vi "ComicCleaner.vi"() -> ()   [LabVIEW 2022 SP3]
uses:
  TypeDefs/Main States.ctl
  TypeDefs/Tag Cmd.ctl
panel:
  in  "Clean Filename?":bool=TRUE
  out "Total":i32
  out "Progress":i32(slide) max=10 scale=0.0..4.0
  out "Current File":string
  in  "Directory":path
  out "Status":string
  out "Crufted Files":string[](array[string])
  in  "Single File":path
  out "Working Folder":path=path "C:/Users/Mark/Documents/Temp"
  in  "Exit":bool
  # "of"
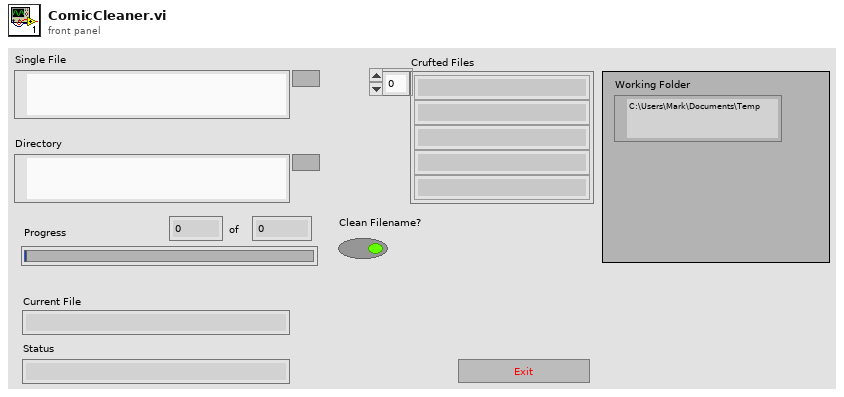
[diagram p1: front panel]
types:
  T1 = typedef "Main States.ctl" = enum16{"Init", "Clean Single", "Clean Dir", "Wait For Input", "Exit"}
  T2 = typedef "Tag Cmd.ctl" = enum16{"Init", "Get Known", "Set Known"}
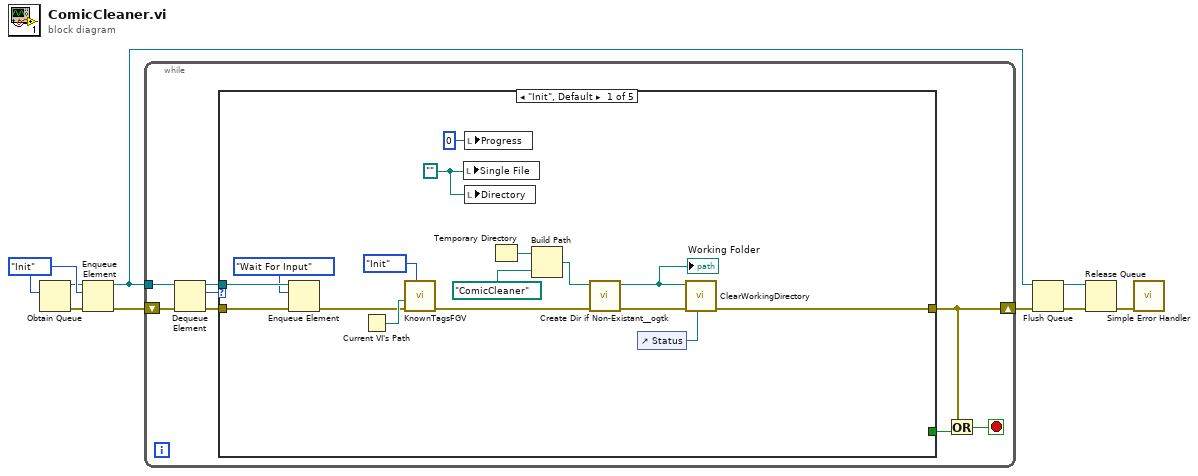
[diagram p0: block diagram]
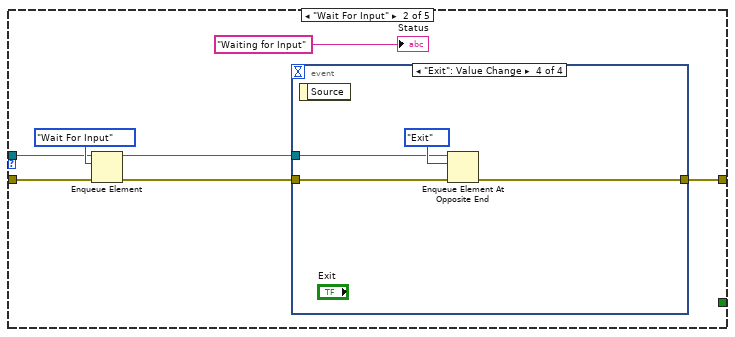
[diagram p2: hidden frame]
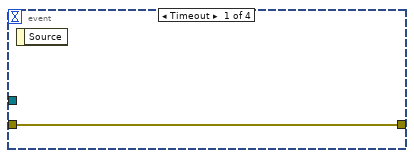
[diagram p3: hidden frame]
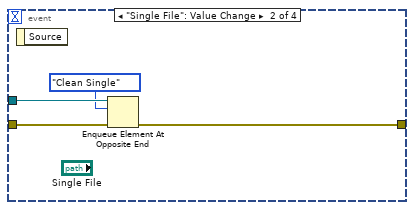
[diagram p4: hidden frame]
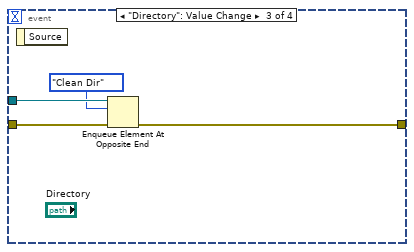
[diagram p5: hidden frame]
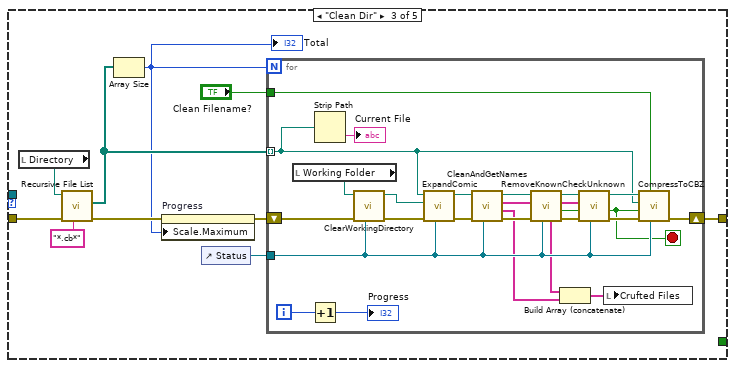
[diagram p6: hidden frame]
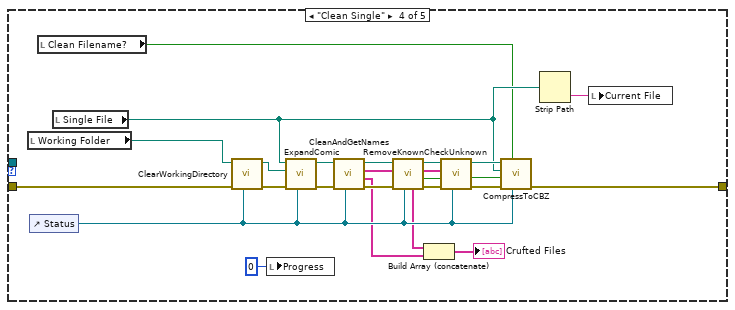
[diagram p7: hidden frame]
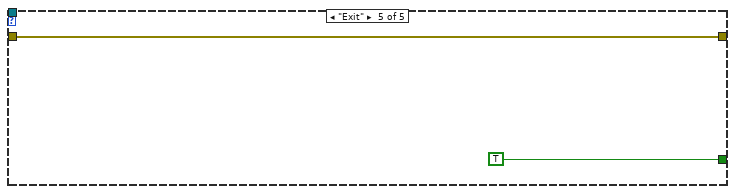
[diagram p8: hidden frame]
diagram:
  w9 = Main_States."Init" ("State")
  n1 = Obtain Queue(element data type=w9) -> (queue out=w8:refnum<queue>, error out=w7:errorcluster)  [unwired: 4 in, 1 out]
  n2 = Enqueue Element(queue=w8, element=w9, error in (no error)=w7) -> (queue out=w1:refnum<queue>, error out=w6:errorcluster)  [unwired: 1 in, 1 out]
  n3 = while {
    shift-right: [w10] -> w3
    shift-left: w6 -> [w17]
    tunnel: w1 -> [w16]
    stop <- w12 stop-if-true
    n4 = Dequeue Element(queue=w16, error in (no error)=w17) -> (queue out=w11:refnum<queue>, element=w15:T1, error out=w14:errorcluster)  [unwired: 1 in, 1 out]
    n5 = case shown="\"Init\", Default" w15 {
      tunnel: w11 -> [w29 w37 _ _ _]
      tunnel: w14 -> [w28 w36 w63 w114 w115]
      tunnel: [_ _ _ _ TRUE] -> w13
      tunnel: [w30 w40 w60 w99 w115] -> w10
      frame "Init", Default {
        w24 = path ""
        n6 = Enqueue Element(queue=w29, element=Main_States."Wait For Input" ("State"), error in (no error)=w28) -> (error out=w27:errorcluster)  [unwired: 1 in, 2 out]
        n7 = Current VI's Path() -> (path=w32:path)
        n8 = call "KnownTagsFGV.vi"("Tag Cmd"=Tag_Cmd."Init", "error in (no error)"=w27, "ini Path"=w32) -> ("error out"=w20:errorcluster)  [unwired: 7 in, 1 out]
        n9 = local write "Single File"(w24) -> ()
        n10 = local write "Progress"(u8 0 ("Progress")) -> ()
        n11 = local write "Directory"(w24) -> ()
        n12 = Temporary Directory() -> (w23:path)
        n13 = Build Path(base path=w23, name or relative path=path "ComicCleaner") -> (appended path=w21:path)
        n14 = call <userlib>:"Create Dir if Non-Existant__ogtk.vi"("error in (no error)"=w20, "Directory Path"=w21) -> ("error out"=w19:errorcluster, "dup Directory Path"=w18:path)  [unwired: 7 in, 1 out]
        "Working Folder" <- w18
        n15 = control-ref of="Status"() -> (w31:refnum<vi>)
        n16 = call "ClearWorkingDirectory.vi"("Status"=w31, "error in"=w19, "Working Path"=w18) -> ("error out"=w30:errorcluster)  [unwired: 7 in, 1 out]
      }
      frame "Wait For Input" {
        n17 = Enqueue Element(queue=w37, element=Main_States."Wait For Input" ("State"), error in (no error)=w36) -> (queue out=w34:refnum<queue>, error out=w35:errorcluster)  [unwired: 1 in, 1 out]
        n18 = event shown="[3] \"Exit\": Value Change" {
          selector: _ -> [_ _ _ _]
          dyn-events: _ -> [_ _ _ _]
          timeout: _ -> [_ _ _ _]
          tunnel: [w41 w42 w46 w50] -> w40
          tunnel: w35 -> [w41 w45 w49 w51]
          tunnel: w34 -> [_ w44 w48 w52]
          event Timeout {
            n19 = event-data() -> ()  [unwired: 1 in, 1 out]
          }
          event "Single File": Value Change {
            n20 = event-data() -> ()  [unwired: 1 in, 1 out]
            n21 = Enqueue Element At Opposite End(queue=w44, element=Main_States."Clean Single" ("State"), error in (no error)=w45) -> (error out=w42:errorcluster)  [unwired: 1 in, 2 out]
          }
          event "Directory": Value Change {
            n22 = event-data() -> ()  [unwired: 1 in, 1 out]
            n23 = Enqueue Element At Opposite End(queue=w48, element=Main_States."Clean Dir" ("State"), error in (no error)=w49) -> (error out=w46:errorcluster)  [unwired: 1 in, 2 out]
          }
          event "Exit": Value Change {
            n24 = event-data() -> ()  [unwired: 1 in, 1 out]
            n25 = Enqueue Element At Opposite End(queue=w52, element=Main_States."Exit" ("State"), error in (no error)=w51) -> (error out=w50:errorcluster)  [unwired: 1 in, 2 out]
          }
        }
        "Status" <- "Waiting for Input" ("Status")
      }
      frame "Clean Dir" {
        n26 = local read "Directory"() -> (w62:path)
        n27 = call <vilib>:"Recursive File List.vi"("pattern"="*.cb*", "error in (no error)"=w63, "Folder Path"=w62) -> ("error out"=w57:errorcluster, "All Files in Dir"=w58:path[])  [unwired: 4 in, 3 out]
        n28 = Array Size(array=w58) -> (size(s)=w55:i32)
        "Total" <- w55
        n29 = property on="Progress" class="Slide (strict)"(error in=w57, "Scale.Maximum"=w55) -> (error out=w56:errorcluster)  [unwired: 1 in, 1 out]
        n30 = control-ref of="Status"() -> (w59:refnum<vi>)
        n31 = for {
          N: w55 -> [_]
          shift-right: [w73] -> w60
          shift-left: w56 -> [w74]
          tunnel: w58 -> [w72] mode=indexing
          tunnel: w59 -> [w75]
          tunnel: "Clean Filename?" -> [w64]
          i -> [w66]
          stop <- w70 stop-if-true
          n32 = local read "Working Folder"() -> (w89:path)
          n33 = Increment(x=w66) -> (x+1=→"Progress":i32)
          n34 = Strip Path(path=w72) -> (name=→"Current File":string)  [unwired: 1 out]
          n35 = call "ClearWorkingDirectory.vi"("Status"=w75, "error in"=w74, "Working Path"=w89) -> ("error out"=w88:errorcluster, "Working Path Out"=w87:path)  [unwired: 7 in]
          n36 = call "ExpandComic.vi"("Status"=w75, "error in (no error)"=w88, "Working Dir"=w87, "Source"=w72) -> ("error out"=w85:errorcluster, "Working Dir Out"=w86:path)  [unwired: 6 in]
          n37 = call "CleanAndGetNames.vi"("Status"=w75, "error in"=w85, "Working Dir"=w86) -> ("error out"=w84:errorcluster, "Deleted files"=w68:string[], "filenames"=w83:string[], "Working Dir Out"=w82:path)  [unwired: 5 in]
          n38 = call "RemoveKnown.vi"("Status"=w75, "error in (no error)"=w84, "filenames"=w83, "Working Dir"=w82) -> ("error out"=w80:errorcluster, "Known Found?"=w79:bool, "Filenames Out"=w78:string[], "Working Dir Out"=w81:path, "Tags Removed"=w69:string[])  [unwired: 3 in]
          n39 = Build Array (concatenate)(w69, w68) -> (w67:string[])
          n40 = call "CheckUnknown.vi"("Status"=w75, "error in (no error)"=w80, "Known Found?"=w79, "filenames"=w78, "Working Dir"=w81) -> ("error out"=w76:errorcluster, "Abort?"=w70:bool, "Working Dir Out"=w77:path)  [unwired: 4 in]
          n41 = local write "Crufted Files"(w67) -> ()
          n42 = call "CompressToCBZ.vi"("Status"=w75, "Clean Filename?"=w64, "error in"=w76, "Abort?"=w70, "FormerFilename"=w72, "Working Path"=w77) -> ("error out"=w73:errorcluster)  [unwired: 4 in, 1 out]
        }
      }
      frame "Clean Single" {
        n43 = local read "Working Folder"() -> (w113:path)
        n44 = control-ref of="Status"() -> (w98:refnum<vi>)
        n45 = local read "Clean Filename?"() -> (w90:bool)
        n46 = local read "Single File"() -> (w97:path)
        n47 = call "ClearWorkingDirectory.vi"("Status"=w98, "error in"=w114, "Working Path"=w113) -> ("error out"=w112:errorcluster, "Working Path Out"=w111:path)  [unwired: 7 in]
        n48 = local write "Progress"(u8 0 ("Progress")) -> ()
        n49 = call "ExpandComic.vi"("Status"=w98, "error in (no error)"=w112, "Working Dir"=w111, "Source"=w97) -> ("error out"=w109:errorcluster, "Working Dir Out"=w110:path)  [unwired: 6 in]
        n50 = call "CleanAndGetNames.vi"("Status"=w98, "error in"=w109, "Working Dir"=w110) -> ("error out"=w108:errorcluster, "Deleted files"=w93:string[], "filenames"=w107:string[], "Working Dir Out"=w106:path)  [unwired: 5 in]
        n51 = call "RemoveKnown.vi"("Status"=w98, "error in (no error)"=w108, "filenames"=w107, "Working Dir"=w106) -> ("error out"=w104:errorcluster, "Known Found?"=w103:bool, "Filenames Out"=w102:string[], "Working Dir Out"=w105:path, "Tags Removed"=w94:string[])  [unwired: 3 in]
        n52 = Build Array (concatenate)(w94, w93) -> (→"Crufted Files":string[])
        n53 = call "CheckUnknown.vi"("Status"=w98, "error in (no error)"=w104, "Known Found?"=w103, "filenames"=w102, "Working Dir"=w105) -> ("error out"=w100:errorcluster, "Abort?"=w95:bool, "Working Dir Out"=w101:path)  [unwired: 4 in]
        n54 = call "CompressToCBZ.vi"("Status"=w98, "Clean Filename?"=w90, "error in"=w100, "Abort?"=w95, "FormerFilename"=w97, "Working Path"=w101) -> ("error out"=w99:errorcluster)  [unwired: 4 in, 1 out]
        n55 = Strip Path(path=w97) -> (name=w96:string)  [unwired: 1 out]
        n56 = local write "Current File"(w96) -> ()
      }
      frame "Exit" {
      }
    }
    n57 = Or(x=w10, y=w13) -> (x .or. y?=w12:bool)
  }
  n58 = Flush Queue(queue=w1, error in (no error)=w3) -> (queue out=w5:refnum<queue>, error out=w4:errorcluster)  [unwired: 1 out]
  n59 = Release Queue(queue=w5, error in (no error)=w4) -> (error out=w2:errorcluster)  [unwired: 1 in, 2 out]
  n60 = call <vilib>:"Simple Error Handler.vi"("error in (no error)"=w2) -> ()  [unwired: 4 in, 5 out]
